vi "CODMn通讯.vi"() -> ()   [LabVIEW 2016, in "斯坦道CODMn.lvlib"]
uses:
  <vilib>/NI/Modbus Library/API/Wrapper/Create TCP Slave.vi
  <vilib>/NI/Modbus Library/API/slave/Modbus Slave.lvclass
  <vilib>/Plasmionique/MB Master/MB_Master/MB_Master.lvclass
  <vilib>/Plasmionique/MB Master/MB Master.lvlib
  <vilib>/Utility/config.llb/NI_LVConfig.lvlib
  <vilib>/NI/Modbus Library/API/Wrapper/API Main.lvlib
panel:
  in  "读取数据":bool
  in  "释放串口":bool
  in  "打开串口":bool
  out "队列中元素数量":i32
  out "元素":cluster{"命令":string}[](array[cluster])
  out "待处理插入数量":i32
  out "读取公式":u16[](array[numeric])
  out "读取参数":u16[](array[numeric])
  out "数据存储":u16[](array[numeric])
  out "温度":bool[](array[boolean])
  out "M输出点":bool[](array[boolean])
  out "ORP、时间":u16[](array[numeric])
  out "测量状态":u16[](array[numeric])
  out "通讯状态":bool
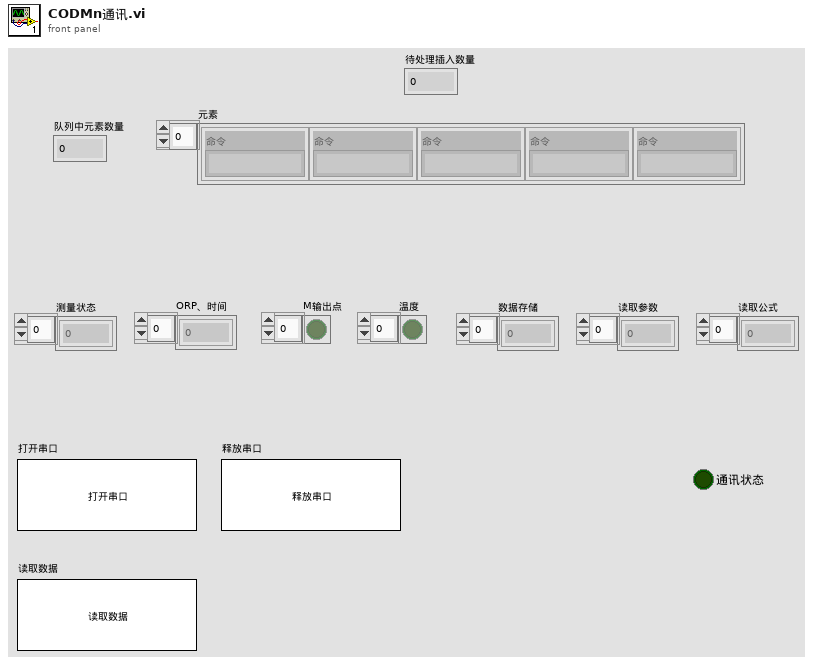
[diagram p1: front panel]
types:
  T1 = cluster{"测量模式":enum16{"水样测量", "标样核查", "零点核查", "跨度核查", "空白测试", "加标回收", "平行样", "校零", "校标"}}
  T2 = cluster{"命令":string, "测量模式":enum16{"水样测量", "标样核查", "零点核查", "跨度核查", "空白测试", "加标回收", "平行样", "校零", "校标"}, "CODMn量程切换":enum32{"H", "L", "AUTO"}}
  T3 = typedef "NI_LVConfig.lvlib/Config Data RefNum.ctl" = refnum<k1>
  T4 = enum16{"空闲", "水样测试", "标样核查", "零点核查", "跨度核查", "空白测试", "平行样测试", "质控样", "空白校准", "标样校准", "加标回收"}
  T5 = enum16{"水样测量", "标样核查", "零点核查", "跨度核查", "空白测试", "加标回收", "平行样", "校零", "校标"}
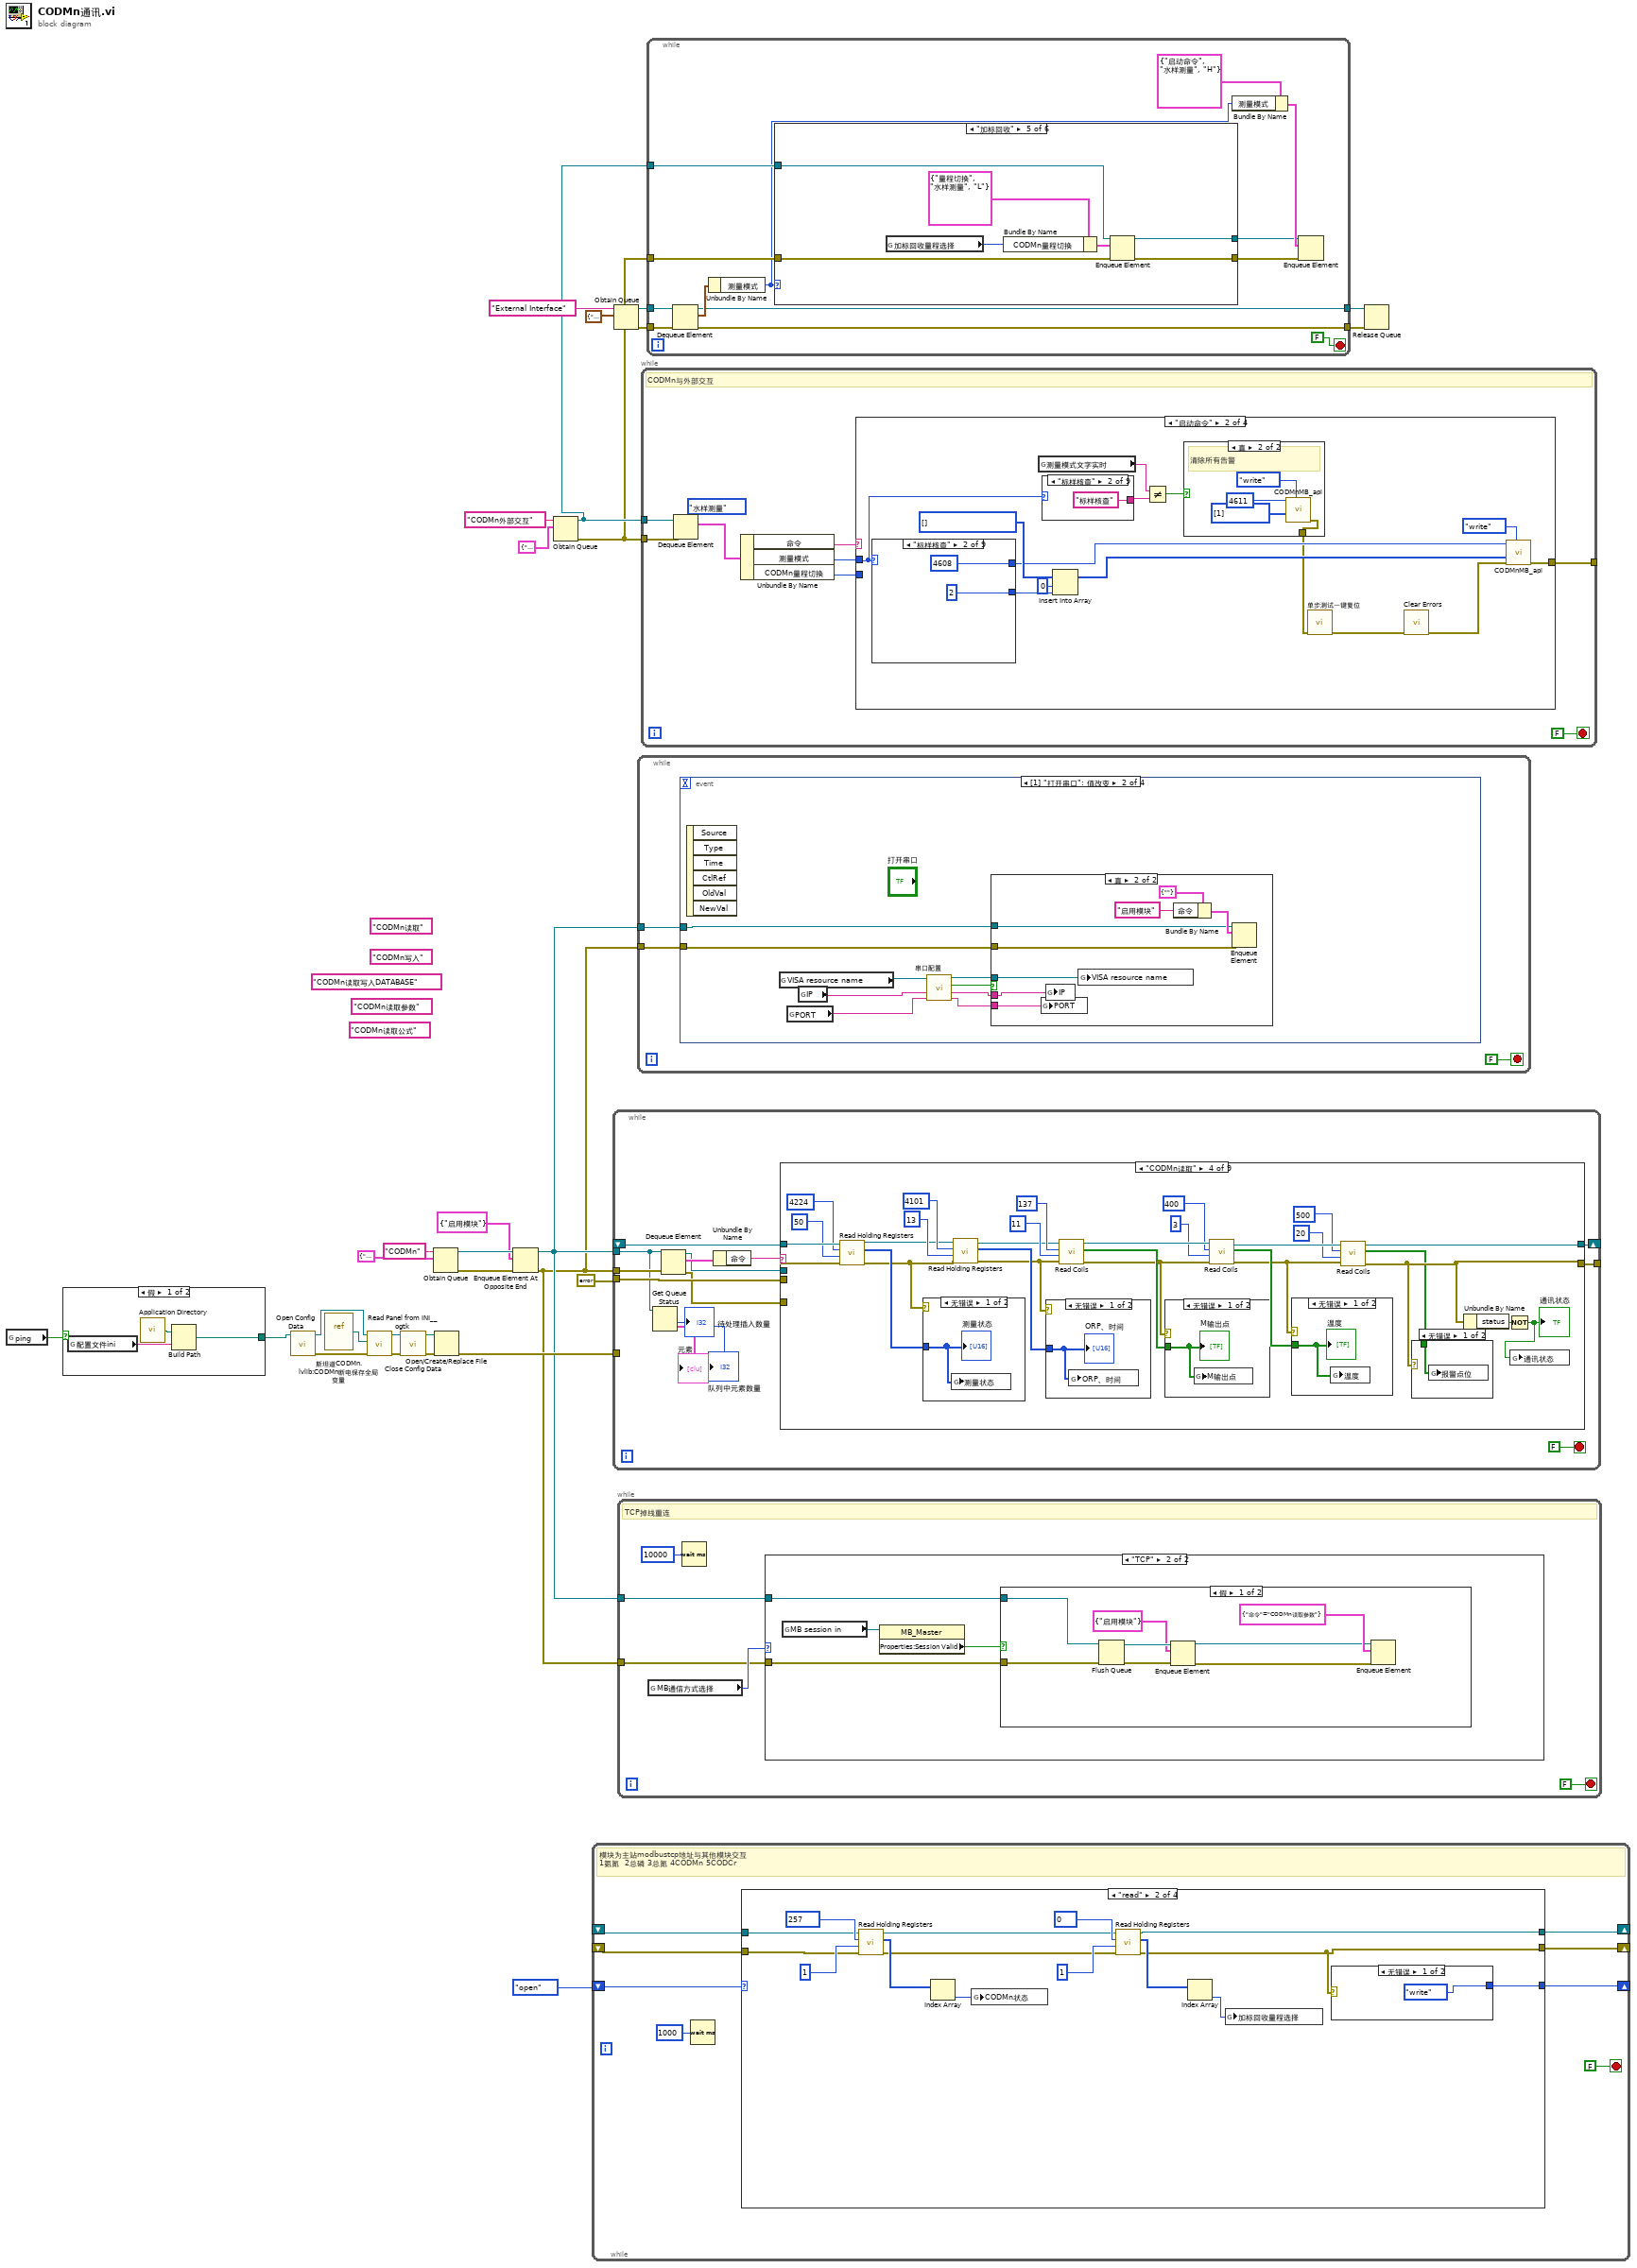
[diagram p0: block diagram]
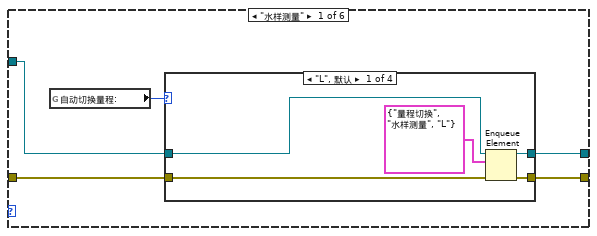
[diagram p2: hidden frame]
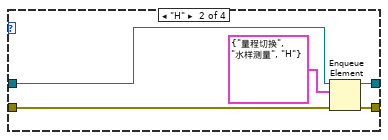
[diagram p3: hidden frame]
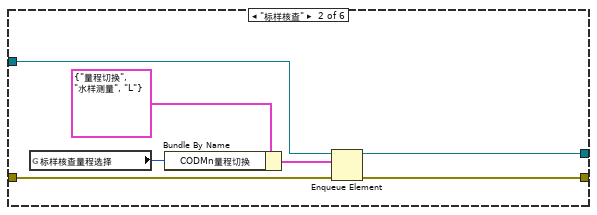
[diagram p6: hidden frame]
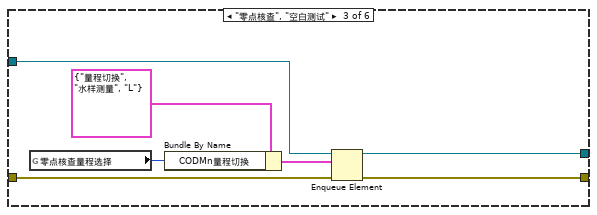
[diagram p7: hidden frame]
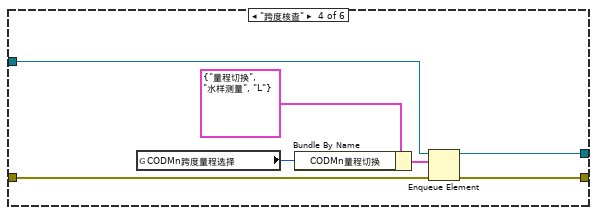
[diagram p8: hidden frame]
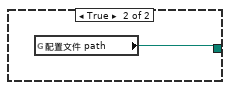
[diagram p10: hidden frame]
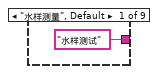
[diagram p13: hidden frame]
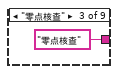
[diagram p14: hidden frame]
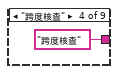
[diagram p15: hidden frame]
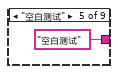
[diagram p16: hidden frame]
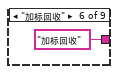
[diagram p17: hidden frame]
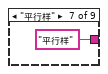
[diagram p18: hidden frame]
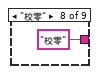
[diagram p19: hidden frame]
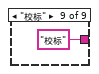
[diagram p20: hidden frame]
diagram:
  (unwired) "CODMn读取公式" ("名称（未命名）")
  (unwired) "CODMn读取写入DATABASE" ("名称（未命名）")
  (unwired) "CODMn读取参数" ("名称（未命名）")
  (unwired) "CODMn读取" ("名称（未命名）")
  (unwired) "CODMn写入" ("名称（未命名）")
  n1 = global read "CODMN外部API.vi" "ping"() -> (w10:bool)
  n2 = case shown="假" w10 {
    tunnel: [w30 w33] -> w9
    frame False {
      n3 = global read "COD内部交互全局.vi" "配置文件ini"() -> (w32:string)
      n4 = call <vilib>:"Application Directory.vi"() -> ("Application Directory"=w31:path)
      n5 = Build Path(base path=w31, name or relative path=w32) -> (appended path=w30:path)
    }
    frame True {
      n6 = global read "CODMN外部API.vi" "配置文件 path"() -> (w33:path)
    }
  }
  n7 = call <vilib>:"Open Config Data.vi"("configuration file path"=w9) -> ("error out"=w20:errorcluster, "refnum"=w23:T3)  [unwired: 8 in, 1 out]
  n8 = vi-ref "斯坦道CODMn.lvlib:CODMn断电保存全局变量.vi"() -> (w22:refnum<vi>)
  n9 = call <userlib>:"Read Panel from INI__ogtk.vi"("error in (no error)"=w20, "VI ref"=w22, "refnum"=w23) -> ("error out"=w19:errorcluster, "refnum out"=w21:T3)  [unwired: 7 in]
  n10 = call <vilib>:"Close Config Data.vi"("error in (no error)"=w19, "refnum"=w21) -> ("error out"=w18:errorcluster, "file path"=w17:path)  [unwired: 8 in]
  n11 = Obtain Queue(name (unnamed)="CODMn" ("名称（未命名）"), element data type=cluster{"命令":string} {"命令"="启用模块"} ("元素")) -> (queue out=w26:refnum<queue>, error out=w25:errorcluster)  [unwired: 3 in, 1 out]
  n12 = Open/Create/Replace File(file path (use dialog)=w17, error in=w18) -> (error out=w16:errorcluster)  [unwired: 4 in, 2 out]
  n13 = Enqueue Element At Opposite End(queue=w26, element=cluster{"命令":string} {"命令"="启用模块"} ("元素"), error in (no error)=w25) -> (queue out=w14:refnum<queue>, error out=w13:errorcluster)  [unwired: 1 in, 1 out]
  n14 = Obtain Queue(name (unnamed)="CODMn外部交互" ("名称（未命名）"), element data type=T2 {"命令"="启动命令", "测量模式"=enum."水样测量", "CODMn量程切换"=enum."AUTO"} ("元素")) -> (queue out=w4:refnum<queue>, error out=w3:errorcluster)  [unwired: 3 in, 1 out]
  n15 = while {
    shift-right: [w39] -> _
    shift-left: _ -> [w41]
    shift-right: [w38] -> _
    shift-left: _ -> [w40]
    shift-right: [w35] -> _
    shift-left: enum16{"open", "read", "write", "close"}."open" -> [w36]
    stop <- FALSE stop-if-true
    # "模块为主站modbustcp地址与其他模块交互\n1氨氮  2总磷 3总氮 4CODMn 5CODCr"
    n16 = Wait (ms)(milliseconds to wait=u32 1000 ("等待时间（毫秒）")) -> ()  [unwired: 1 out]
    n17 = case shown="\"read\"" w36 {
      selector: w36 -> [w50 _ _ _]
      tunnel: w41 -> [w44 w64 w87 w93]
      tunnel: w40 -> [w43 w63 w84 w92]
      tunnel: [w47 w55 w86 w93] -> w39
      tunnel: [w46 w54 w85 w95] -> w38
      tunnel: [w49 w67 w88 enum16{"open", "read", "write", "close"}."open"] -> w35
      frame "open", Default {
        n18 = call-dynamic "Shutdown.vi"("error in"=w43, "Modbus slave in"=w44) -> ("error out"=w42:errorcluster)  [unwired: 9 in]
        n19 = call <vilib>:"Clear Errors.vi"("error in (no error)"=w42) -> ("error out"=w45:errorcluster)  [unwired: 5 in, 1 out]
        n20 = call-poly <vilib>:"Create Modbus Instance.vi"("error in"=w45, "port (502)"=u16 4) -> ("error out"=w46:errorcluster, "TCP slave instance"=w47:refnum<class "Modbus Slave.lvclass">)  [unwired: 8 in]
        n21 = case shown="错误" w46 {
          tunnel: w50 -> [_ w52]
          tunnel: [enum16{"open", "read", "write", "close"}."write" w52] -> w49
          frame No Error {
          }
          frame Error {
          }
        }
      }
      frame "read" {
        n22 = call-dynamic <vilib>:"Read Holding Registers.vi"("error in"=w63, "number of inputs"=u16 1, "starting address"=u16 257, "Modbus slave in"=w64) -> ("error out"=w56:errorcluster, "register values"=w62:u16[], "Modbus slave out"=w57:refnum<class "Modbus Slave.lvclass">)  [unwired: 5 in]
        n23 = Index Array(array=w62) -> (element=w61:u16)  [unwired: 1 in]
        n24 = global write "CODMN外部API.vi" "CODMn状态"(w61) -> ()
        n25 = call-dynamic <vilib>:"Read Holding Registers.vi"("error in"=w56, "number of inputs"=u16 1, "starting address"=u16 0, "Modbus slave in"=w57) -> ("error out"=w54:errorcluster, "register values"=w60:u16[], "Modbus slave out"=w55:refnum<class "Modbus Slave.lvclass">)  [unwired: 5 in]
        n26 = Index Array(array=w60) -> (element=w53:u16)  [unwired: 1 in]
        n27 = global write "CODMn断电保存全局变量.vi" "加标回收量程选择"(w53) -> ()
        n28 = case shown="无错误" w54 {
          tunnel: [enum16{"open", "read", "write", "close"}."write" enum16{"open", "read", "write", "close"}."close"] -> w67
          frame No Error {
          }
          frame Error {
          }
        }
      }
      frame "write" {
        n29 = global read "COD测量模式全局.vi" "CODMn工作状态"() -> (w74:T4)
        n30 = global read "COD浓度全局变量.vi" "COD浓度（mg/L)"() -> (w76:dbl)
        n31 = global read "COD测量模式全局.vi" "加标回收启动时间"() -> (w79:timestamp)
        n32 = global read "COD测量模式全局.vi" "水样启动时间"() -> (w81:timestamp)
        n33 = global read "运行时序全局变量.vi" "多列列表框"() -> (w78:i32)
        n34 = Build Array(w81) -> (w80:timestamp[])
        n35 = Build Array(w76) -> (w75:dbl[])
        n36 = Build Array(w79) -> (w72:timestamp[])
        n37 = call "浮点转CDAB整形cod.vi"("浮点数"=w75) -> ("CDAB整形输出"=w77:u16[])  [unwired: 10 in]
        n38 = call "DateToHex.vi"("DATE"=w80) -> ("数组"=w83:u16[])  [unwired: 10 in]
        n39 = call "DateToHex.vi"("DATE"=w72) -> ("数组"=w82:u16[])  [unwired: 10 in]
        n40 = Insert Into Array(array=u16[] [] ("values"), new element #1=w74, new element #2=w77, new element #3=w78, new element #4=w82, new element #5=w83) -> (w71:u16[])  [unwired: 1 in]
        n41 = call-dynamic "Write Multiple Holding Registers.vi"("error in"=w84, "registers to write"=w71, "starting address"=u16 0, "Modbus slave in"=w87) -> ("error out"=w85:errorcluster, "Modbus slave out"=w86:refnum<class "Modbus Slave.lvclass">)  [unwired: 6 in]
        n42 = case shown="无错误" w85 {
          tunnel: [enum16{"open", "read", "write", "close"}."read" enum16{"open", "read", "write", "close"}."close"] -> w88
          frame No Error {
          }
          frame Error {
          }
        }
      }
      frame "close" {
        n43 = call-dynamic "Shutdown.vi"("error in"=w92, "Modbus slave in"=w93) -> ("error out"=w91:errorcluster)  [unwired: 9 in]
        n44 = call <vilib>:"Clear Errors.vi"("error in (no error)"=w91) -> ("error out"=w95:errorcluster)  [unwired: 5 in, 1 out]
      }
    }
  }
  n45 = while {
    tunnel: w14 -> [w101]
    tunnel: w13 -> [w108]
    tunnel: [w102] -> _
    shift-right: [w105] -> _
    shift-left: _ -> [w104]
    tunnel: errorcluster {"status"=FALSE, "code"=0, "source"=""} ("error out") -> [w103]
    tunnel: w16 -> [_]
    stop <- FALSE stop-if-true
    n46 = Get Queue Status(queue=w101) -> (# pending insert=→"待处理插入数量":i32, # elements in queue=→"队列中元素数量":i32, elements=→"元素":cluster{"命令":string}[])  [unwired: 2 in, 5 out]
    n47 = Dequeue Element(queue=w101, error in (no error)=w108) -> (queue out=w97:refnum<queue>, element=w107:cluster{"命令":string}, error out=w96:errorcluster)  [unwired: 1 in, 1 out]
    n48 = Unbundle By Name(w107) -> ("命令"=w106:string)
    n49 = case shown="\"CODMn读取\"" w106 {
      tunnel: [w111 w115 w126 w134 w166 w175 w192 w199 w206] -> w105
      tunnel: [w110 w112 w127 w131 w164 w174 w191 w198 w205] -> w102
      tunnel: w104 -> [w111 _ _ w158 w170 w184 w195 w203 w209]
      tunnel: w103 -> [w110 w116 w128 w157 w167 w183 w194 w202 w207]
      tunnel: w97 -> [_ w114 _ _ _ _ _ _ _]
      tunnel: w96 -> [_ w113 _ _ _ _ _ _ _]
      frame Default {
      }
      frame "启用模块" {
        n50 = call "CODMnMB_api.vi"("STEP"=enum16{"open", "read", "write", "close"}."open", "Error in"=w116) -> ("error out"=w112:errorcluster, "MB session out"=w115:refnum<class "MB_Master.lvclass">)  [unwired: 7 in, 1 out]
        n51 = case shown="无错误" w112 {
          tunnel: w114 -> [w122 _]
          tunnel: w113 -> [w121 _]
          frame No Error {
            n52 = global read "COD内部交互全局.vi" "序列号:"() -> (w120:string)
            n53 = Empty String/Path?(string/path=w120) -> (empty?=w119:bool)
            n54 = Not(x=w119) -> (.not. x?=w118:bool)
            n55 = case shown="真" w118 {
              tunnel: w122 -> [_ w125]
              tunnel: w121 -> [_ w124]
              frame False {
              }
              frame True {
                # "发货调试版用"
                n56 = Enqueue Element(queue=w125, element=cluster{"命令":string} {"命令"="CODMn序列号写入"} ("元素"), error in (no error)=w124) -> ()  [unwired: 1 in, 3 out]
              }
            }
          }
          frame Error {
          }
        }
        n57 = global write "COD浓度全局变量.vi" "MB session in"(w115) -> ()
      }
      frame "停用模块" {
        n58 = call "CODMnMB_api.vi"("STEP"=enum16{"open", "read", "write", "close"}."close", "Error in"=w128) -> ("error out"=w127:errorcluster, "MB session out"=w126:refnum<class "MB_Master.lvclass">)  [unwired: 7 in, 1 out]
      }
      frame "CODMn读取" {
        n59 = call <vilib>:"Read Holding Registers.vi"("error in (no error)"=w157, "quantity"=u16 50 ("number of holding registers"), "starting address"=u16 4224, "MB session in"=w158) -> ("error out"=w148:errorcluster, "Registers"=w154:u16[], "MB session out"=w149:refnum<class "MB_Master.lvclass">)  [unwired: 5 in]
        n60 = case shown="无错误" w148 {
          tunnel: w154 -> [w163 _]
          frame No Error {
            n61 = global write "COD内部交互全局.vi" "测量状态"(w163) -> ()
            "测量状态" <- w163
          }
          frame Error {
          }
        }
        n62 = call <vilib>:"Read Holding Registers.vi"("error in (no error)"=w148, "quantity"=u16 13, "starting address"=u16 4101, "MB session in"=w149) -> ("error out"=w144:errorcluster, "Registers"=w147:u16[], "MB session out"=w146:refnum<class "MB_Master.lvclass">)  [unwired: 5 in]
        n63 = case shown="无错误" w144 {
          tunnel: w147 -> [w162 _]
          frame No Error {
            n64 = global write "COD内部交互全局.vi" "ORP、时间"(w162) -> ()
            "ORP、时间" <- w162
          }
          frame Error {
          }
        }
        n65 = call <vilib>:"Read Coils.vi"("error in (no error)"=w144, "quantity"=u16 11, "starting address"=u16 137, "MB session in"=w146) -> ("error out"=w142:errorcluster, "Coils"=w143:bool[], "MB session out"=w145:refnum<class "MB_Master.lvclass">)  [unwired: 5 in]
        n66 = case shown="无错误" w142 {
          tunnel: w143 -> [w161 _]
          frame No Error {
            n67 = global write "COD内部交互全局.vi" "M输出点"(w161) -> ()
            "M输出点" <- w161
          }
          frame Error {
          }
        }
        n68 = call <vilib>:"Read Coils.vi"("error in (no error)"=w142, "quantity"=u16 3, "starting address"=u16 400, "MB session in"=w145) -> ("error out"=w135:errorcluster, "Coils"=w139:bool[], "MB session out"=w136:refnum<class "MB_Master.lvclass">)  [unwired: 5 in]
        n69 = case shown="无错误" w135 {
          tunnel: w139 -> [w160 _]
          frame No Error {
            n70 = global write "COD内部交互全局.vi" "温度"(w160) -> ()
            "温度" <- w160
          }
          frame Error {
          }
        }
        n71 = call <vilib>:"Read Coils.vi"("error in (no error)"=w135, "quantity"=u16 20, "starting address"=u16 500, "MB session in"=w136) -> ("error out"=w131:errorcluster, "Coils"=w130:bool[], "MB session out"=w134:refnum<class "MB_Master.lvclass">)  [unwired: 5 in]
        n72 = case shown="无错误" w131 {
          tunnel: w130 -> [w159 _]
          frame No Error {
            n73 = global write "COD内部交互全局.vi" "报警点位"(w159) -> ()
          }
          frame Error {
          }
        }
        n74 = Unbundle By Name(w131) -> ("status"=w138:bool)
        n75 = Not(x=w138) -> (.not. x?=w137:bool)
        "通讯状态" <- w137
        n76 = global write "COD内部交互全局.vi" "通讯状态"(w137) -> ()
      }
      frame "CODMn读取写入DATABASE" {
        n77 = call <vilib>:"Read Holding Registers.vi"("error in (no error)"=w167, "quantity"=u16 10 ("number of holding registers"), "starting address"=u16 4101, "MB session in"=w170) -> ("error out"=w164:errorcluster, "Registers"=w165:u16[], "MB session out"=w166:refnum<class "MB_Master.lvclass">)  [unwired: 5 in]
        n78 = case shown="无错误" w164 {
          tunnel: w165 -> [w172 _]
          frame No Error {
            n79 = global write "COD内部交互全局.vi" "数据存储"(w172) -> ()
            n80 = global write "COD内部交互全局.vi" "读取写入data"(TRUE ("读取参数显示")) -> ()
            "数据存储" <- w172
          }
          frame Error {
          }
        }
      }
      frame "CODMn读取参数" {
        n81 = call <vilib>:"Read Holding Registers.vi"("error in (no error)"=w183, "quantity"=u16 35 ("number of holding registers"), "starting address"=u16 4272, "MB session in"=w184) -> ("error out"=w178:errorcluster, "Registers"=w180:u16[], "MB session out"=w179:refnum<class "MB_Master.lvclass">)  [unwired: 5 in]
        n82 = case shown="无错误" w178 {
          tunnel: w180 -> [w188 _]
          frame No Error {
            n83 = global write "COD内部交互全局.vi" "读取参数"(w188) -> ()
            n84 = global write "COD内部交互全局.vi" "读取参数显示"(TRUE ("读取参数显示")) -> ()
            "读取参数" <- w188
          }
          frame Error {
          }
        }
        n85 = call <vilib>:"Read Holding Registers.vi"("error in (no error)"=w178, "quantity"=u16 4, "starting address"=u16 5596, "MB session in"=w179) -> ("error out"=w174:errorcluster, "Registers"=w173:u16[], "MB session out"=w175:refnum<class "MB_Master.lvclass">)  [unwired: 5 in]
        n86 = case shown="无错误" w174 {
          tunnel: w173 -> [w186 _]
          frame No Error {
            n87 = global write "COD内部交互全局.vi" "读取浮台参数"(w186) -> ()
            n88 = global write "COD内部交互全局.vi" "读取浮台参数显示"(TRUE ("读取参数显示")) -> ()
          }
          frame Error {
          }
        }
      }
      frame "CODMn读取公式" {
        n89 = call <vilib>:"Read Holding Registers.vi"("error in (no error)"=w194, "quantity"=u16 94 ("number of holding registers"), "starting address"=u16 4616, "MB session in"=w195) -> ("error out"=w191:errorcluster, "Registers"=w193:u16[], "MB session out"=w192:refnum<class "MB_Master.lvclass">)  [unwired: 5 in]
        n90 = case shown="无错误" w191 {
          tunnel: w193 -> [w197 _]
          frame No Error {
            n91 = global write "COD内部交互全局.vi" "读取公式"(w197) -> ()
            n92 = global write "COD内部交互全局.vi" "读取公式显示"(TRUE ("读取参数显示")) -> ()
            "读取公式" <- w197
          }
          frame Error {
          }
        }
      }
      frame "CODMn序列号写入" {
        n93 = global read "COD内部交互全局.vi" "序列号:"() -> (w201:string)
        n94 = call "StringToHex.vi"("STRING"=w201) -> ("数组"=w200:u16[])  [unwired: 10 in]
        n95 = call <vilib>:"Write Multiple Registers.vi"("error in (no error)"=w202, "values"=w200, "starting address"=u16 4298, "MB session in"=w203) -> ("error out"=w198:errorcluster, "MB session out"=w199:refnum<class "MB_Master.lvclass">)  [unwired: 6 in]
      }
      frame "CODMn程序更新" {
        n96 = call <vilib>:"Write Multiple Registers.vi"("error in (no error)"=w207, "values"=u16[] [0], "starting address"=u16 4296, "MB session in"=w209) -> ("error out"=w205:errorcluster, "MB session out"=w206:refnum<class "MB_Master.lvclass">)  [unwired: 6 in]
      }
    }
  }
  n97 = Obtain Queue(name (unnamed)="External Interface" ("名称（未命名）"), element data type=T1 {"测量模式"=enum."水样测量"} ("启动测量模式")) -> (queue out=w6:refnum<queue>, error out=w5:errorcluster)  [unwired: 3 in, 1 out]
  n98 = while "While循环" {
    tunnel: w14 -> [w212]
    tunnel: w13 -> [w211]
    stop <- FALSE stop-if-true
    # "TCP掉线重连"
    n99 = global read "CODMn断电保存全局变量.vi" "MB通信方式选择"() -> (w213:enum16{"串口", "TCP"})
    n100 = Wait (ms)(milliseconds to wait=u32 10000 ("等待时间（毫秒）")) -> ()  [unwired: 1 out]
    n101 = case shown="\"TCP\"" w213 {
      tunnel: w212 -> [_ w217]
      tunnel: w211 -> [_ w216]
      frame "串口", Default {
      }
      frame "TCP" {
        n102 = global read "COD浓度全局变量.vi" "MB session in"() -> (w219:refnum<class "MB_Master.lvclass">)
        n103 = property class="MB_Master"(reference=w219) -> ("Properties:Session Valid"=w218:bool)  [unwired: 1 in, 2 out]
        n104 = case shown="假" w218 {
          tunnel: w217 -> [w224 _]
          tunnel: w216 -> [w223 _]
          frame False {
            n105 = Flush Queue(queue=w224, error in (no error)=w223) -> (queue out=w227:refnum<queue>, error out=w226:errorcluster)  [unwired: 1 out]
            n106 = Enqueue Element(queue=w227, element=cluster{"命令":string} {"命令"="启用模块"} ("元素"), error in (no error)=w226) -> (queue out=w221:refnum<queue>, error out=w220:errorcluster)  [unwired: 1 in, 1 out]
            n107 = Enqueue Element(queue=w221, element=cluster{"命令":string} {"命令"="CODMn读取参数"} ("元素"), error in (no error)=w220) -> ()  [unwired: 1 in, 3 out]
          }
          frame True {
          }
        }
      }
    }
  }
  n108 = while {
    tunnel: w14 -> [w229]
    tunnel: w13 -> [w228]
    stop <- FALSE stop-if-true
    n109 = event shown="[1] \"打开串口\": 值改变" {
      selector: _ -> [_ _ _ _]
      dyn-events: _ -> [_ _ _ _]
      timeout: _ -> [_ _ _ _]
      tunnel: w229 -> [_ w236 w250 w252]
      tunnel: w228 -> [_ w235 w249 w251]
      event Timeout {
        n110 = event-data() -> ()  [unwired: 1 in, 3 out]
      }
      event "打开串口": Value Change {
        n111 = event-data() -> ()  [unwired: 1 in, 6 out]
        n112 = global read "CODMn断电保存全局变量.vi" "VISA resource name"() -> (w239:refnum<visa-resource-name>)
        n113 = global read "CODMn断电保存全局变量.vi" "PORT"() -> (w231:string)
        n114 = global read "CODMn断电保存全局变量.vi" "IP"() -> (w232:string)
        n115 = call "串口配置.vi"("PORT"=w231, "IP"=w232, "请选择串口:"=w239) -> ("PORT 2"=w233:string, "IP 2"=w234:string, "确认 2"=w237:bool, "VISA资源名称 2"=w238:refnum<visa-resource-name>)  [unwired: 4 in, 1 out]
        n116 = case shown="真" w237 {
          tunnel: w238 -> [_ w247]
          tunnel: w236 -> [_ w243]
          tunnel: w235 -> [_ w242]
          tunnel: w234 -> [_ w241]
          tunnel: w233 -> [_ w240]
          frame False {
          }
          frame True {
            n117 = global write "CODMn断电保存全局变量.vi" "PORT"(w240) -> ()
            n118 = global write "CODMn断电保存全局变量.vi" "IP"(w241) -> ()
            n119 = global write "CODMn断电保存全局变量.vi" "VISA resource name"(w247) -> ()
            n120 = Bundle By Name(cluster=cluster{"命令":string} {"命令"=""} ("元素"), "命令"="启用模块" ("名称（未命名）")) -> (w244:cluster{"命令":string})
            n121 = Enqueue Element(queue=w243, element=w244, error in (no error)=w242) -> ()  [unwired: 1 in, 3 out]
          }
        }
      }
      event "释放串口": Value Change {
        n122 = event-data() -> ()  [unwired: 1 in, 6 out]
        n123 = Enqueue Element(queue=w250, element=cluster{"命令":string} {"命令"="停用模块"} ("元素"), error in (no error)=w249) -> ()  [unwired: 1 in, 3 out]
      }
      event "读取数据": Value Change {
        n124 = event-data() -> ()  [unwired: 1 in, 6 out]
        n125 = Enqueue Element(queue=w252, element=cluster{"命令":string} {"命令"="CODMn读取"} ("元素"), error in (no error)=w251) -> ()  [unwired: 1 in, 3 out]
      }
    }
  }
  n126 = while {
    tunnel: w4 -> [w259]
    tunnel: w3 -> [w258]
    tunnel: [w254] -> _
    stop <- FALSE stop-if-true
    (unwired) T5."水样测量" ("测量模式")
    # "CODMn与外部交互"
    n127 = Dequeue Element(queue=w259, error in (no error)=w258) -> (element=w260:T2)  [unwired: 1 in, 3 out]
    n128 = Unbundle By Name(w260) -> ("命令"=w257:string, "测量模式"=w256:T5, "CODMn量程切换"=w255:enum32{"H", "L", "AUTO"})
    n129 = case shown="\"启动命令\"" w257 {
      tunnel: w256 -> [_ w264 _ _]
      tunnel: w255 -> [_ _ _ w314]
      tunnel: [_ w269 w309 w313] -> w254
      frame "假", Default {
      }
      frame "启动命令" {
        n130 = case shown="\"标样核查\"" w264 {
          tunnel: [u16 4608 ("address") u16 4608 ("address") u16 4608 ("address") u16 4608 ("address") u16 4608 ("address") u16 4608 ("address") u16 4608 ("address") u16 4608 ("address") u16 4608 ("address")] -> w271
          tunnel: [u16 1 ("address") u16 2 ("address") u16 3 ("address") u16 4 ("address") u16 5 ("address") u16 7 ("address") u16 6 ("address") u16 8 ("address") u16 9 ("address")] -> w275
          frame "水样测量" {
          }
          frame "标样核查" {
          }
          frame "零点核查" {
          }
          frame "跨度核查" {
          }
          frame "空白测试" {
          }
          frame "加标回收" {
          }
          frame "平行样" {
          }
          frame "校零" {
            n131 = global write "CODMN外部API.vi" "远程反控校零CODMn"(TRUE ("远程反控校准CODMn")) -> ()
          }
          frame "校标" {
            n132 = global write "CODMN外部API.vi" "远程反控校准CODMn"(TRUE ("远程反控校准CODMn")) -> ()
          }
        }
        n133 = global read "COD测量模式全局.vi" "测量模式文字实时"() -> (w265:string)
        n134 = case shown="\"标样核查\"" w264 {
          tunnel: ["水样测试" ("测量模式") "标样核查" ("测量模式") "零点核查" ("测量模式") "跨度核查" ("测量模式") "空白测试" ("测量模式") "加标回收" ("测量模式") "平行样" ("测量模式") "校零" ("测量模式") "校标" ("测量模式")] -> w266
          frame "水样测量", Default {
          }
          frame "标样核查" {
          }
          frame "零点核查" {
          }
          frame "跨度核查" {
          }
          frame "空白测试" {
          }
          frame "加标回收" {
          }
          frame "平行样" {
          }
          frame "校零" {
          }
          frame "校标" {
          }
        }
        n135 = Insert Into Array(array=u16[] [] ("values"), index=0 ("索引"), new element=w275) -> (w270:u16[])
        n136 = Not Equal?(x=w265, y=w266) -> (x != y?=w263:bool)
        n137 = case shown="真" w263 {
          tunnel: [_ w276] -> w262
          frame False {
          }
          frame True {
            # "清除所有告警"
            n138 = call "CODMnMB_api.vi"("STEP"=enum16{"open", "read", "write", "close"}."write", "values"=u16[] [1], "starting address"=u16 4611) -> ("error out"=w276:errorcluster)  [unwired: 6 in, 2 out]
          }
        }
        n139 = call "单步测试一键复位.vi"("Error in"=w262) -> ("error out"=w268:errorcluster)  [unwired: 10 in]
        n140 = call <vilib>:"Clear Errors.vi"("error in (no error)"=w268) -> ("error out"=w267:errorcluster)  [unwired: 5 in, 1 out]
        n141 = call "CODMnMB_api.vi"("STEP"=enum16{"open", "read", "write", "close"}."write", "Error in"=w267, "values"=w270, "starting address"=w271) -> ("error out"=w269:errorcluster)  [unwired: 5 in, 2 out]
      }
      frame "停止命令" {
        n142 = call "CODMnMB_api.vi"("STEP"=enum16{"open", "read", "write", "close"}."write", "values"=u16[] [11], "starting address"=u16 4608) -> ("error out"=w309:errorcluster)  [unwired: 6 in, 2 out]
      }
      frame "量程切换" {
        n143 = case shown="\"H\"" w314 {
          tunnel: [u16[] [1] ("values") u16[] [0] ("values") _] -> w317
          frame "H" {
          }
          frame "L" {
          }
          frame "AUTO", Default {
          }
        }
        n144 = call "CODMnMB_api.vi"("STEP"=enum16{"open", "read", "write", "close"}."write", "values"=w317, "starting address"=u16 4276) -> ("error out"=w313:errorcluster)  [unwired: 6 in, 2 out]
      }
    }
  }
  n145 = while {
    tunnel: w6 -> [w332]
    tunnel: w5 -> [w331]
    tunnel: w4 -> [w328]
    tunnel: w3 -> [w327]
    tunnel: [w321] -> w2
    tunnel: [w320] -> w1
    stop <- FALSE stop-if-true
    n146 = Dequeue Element(queue=w332, error in (no error)=w331) -> (queue out=w321:refnum<queue>, element=w329:T1, error out=w320:errorcluster)  [unwired: 1 in, 1 out]
    n147 = Unbundle By Name(w329) -> ("测量模式"=w324:T5)
    n148 = case "条件结构" shown="\"加标回收\"" w324 {
      tunnel: w328 -> [w336 w355 w362 w369 w376 w381]
      tunnel: w327 -> [w334 w354 w361 w368 w375 w380]
      tunnel: [w335 w353 w360 w367 w374 w381] -> w323
      tunnel: [w333 w352 w359 w366 w373 w380] -> w322
      frame "水样测量" {
        n149 = global read "CODMn断电保存全局变量.vi" "自动切换量程:"() -> (w337:enum16{"L", "H", "自动切换测一次", "自动切换测两次"})
        n150 = case shown="\"L\", 默认" w337 {
          tunnel: w336 -> [w341 w347 w348 w351]
          tunnel: [w339 w346 w348 w351] -> w335
          tunnel: w334 -> [w340 w345 w349 w350]
          tunnel: [w338 w344 w349 w350] -> w333
          frame "L", Default {
            n151 = Enqueue Element(queue=w341, element=T2 {"命令"="量程切换", "测量模式"=enum."水样测量", "CODMn量程切换"=enum."L"} ("元素"), error in (no error)=w340) -> (queue out=w339:refnum<queue>, error out=w338:errorcluster)  [unwired: 1 in, 1 out]
          }
          frame "H" {
            n152 = Enqueue Element(queue=w347, element=T2 {"命令"="量程切换", "测量模式"=enum."水样测量", "CODMn量程切换"=enum."H"} ("元素"), error in (no error)=w345) -> (queue out=w346:refnum<queue>, error out=w344:errorcluster)  [unwired: 1 in, 1 out]
          }
          frame "自动切换测一次" {
          }
          frame "自动切换测两次" {
          }
        }
      }
      frame "标样核查" {
        n153 = global read "CODMn断电保存全局变量.vi" "标样核查量程选择"() -> (w357:enum32{"H", "L", "AUTO"})
        n154 = Bundle By Name(cluster=T2 {"命令"="量程切换", "测量模式"=enum."水样测量", "CODMn量程切换"=enum."L"} ("元素"), "CODMn量程切换"=w357) -> (w358:T2)
        n155 = Enqueue Element(queue=w355, element=w358, error in (no error)=w354) -> (queue out=w353:refnum<queue>, error out=w352:errorcluster)  [unwired: 1 in, 1 out]
      }
      frame "零点核查", "空白测试" {
        n156 = global read "CODMn断电保存全局变量.vi" "零点核查量程选择"() -> (w364:enum32{"H", "L", "AUTO"})
        n157 = Bundle By Name(cluster=T2 {"命令"="量程切换", "测量模式"=enum."水样测量", "CODMn量程切换"=enum."L"} ("元素"), "CODMn量程切换"=w364) -> (w363:T2)
        n158 = Enqueue Element(queue=w362, element=w363, error in (no error)=w361) -> (queue out=w360:refnum<queue>, error out=w359:errorcluster)  [unwired: 1 in, 1 out]
      }
      frame "跨度核查" {
        n159 = global read "CODMn断电保存全局变量.vi" "CODMn跨度量程选择"() -> (w371:enum32{"H", "L", "AUTO"})
        n160 = Bundle By Name(cluster=T2 {"命令"="量程切换", "测量模式"=enum."水样测量", "CODMn量程切换"=enum."L"} ("元素"), "CODMn量程切换"=w371) -> (w370:T2)
        n161 = Enqueue Element(queue=w369, element=w370, error in (no error)=w368) -> (queue out=w367:refnum<queue>, error out=w366:errorcluster)  [unwired: 1 in, 1 out]
      }
      frame "加标回收" {
        n162 = global read "CODMn断电保存全局变量.vi" "加标回收量程选择"() -> (w378:enum32{"H", "L", "AUTO"})
        n163 = Bundle By Name(cluster=T2 {"命令"="量程切换", "测量模式"=enum."水样测量", "CODMn量程切换"=enum."L"} ("元素"), "CODMn量程切换"=w378) -> (w377:T2)
        n164 = Enqueue Element(queue=w376, element=w377, error in (no error)=w375) -> (queue out=w374:refnum<queue>, error out=w373:errorcluster)  [unwired: 1 in, 1 out]
      }
      frame Default {
        # "不切换量程"
      }
    }
    n165 = Bundle By Name(cluster=T2 {"命令"="启动命令", "测量模式"=enum."水样测量", "CODMn量程切换"=enum."H"} ("元素"), "测量模式"=w324) -> (w325:T2)
    n166 = Enqueue Element(queue=w323, element=w325, error in (no error)=w322) -> ()  [unwired: 1 in, 3 out]
  }
  n167 = Release Queue(queue=w2, error in (no error)=w1) -> ()  [unwired: 1 in, 3 out]
